vi "SA_EN_NON-STD_MEAS.vi"(6 "?":i32(ring) items=["NO", "YES"], 8 "error in":errorcluster {"code" format="%.0x"}, 11 "Session In":refnum<visa-resource-name>="TCPIP0::K-N90X0A-00005.local::hislip0::INSTR") -> (0 "error out":errorcluster {"code" format="%.0x"}, 3 "Session Out":refnum<visa-resource-name>)   [LabVIEW 2018]
panel:
  out "concatenated string":string
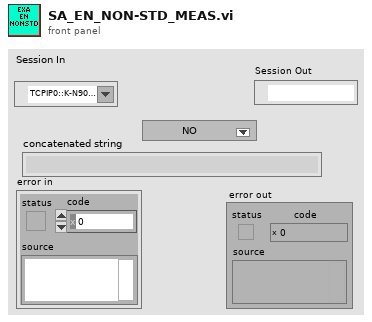
[diagram p1: front panel]
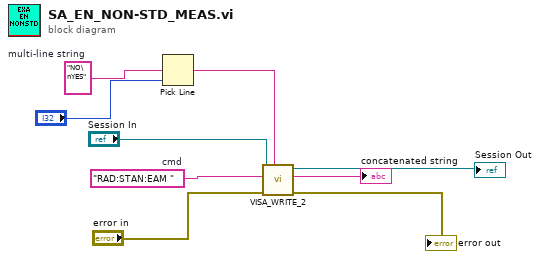
[diagram p0: block diagram]
diagram:
  w3 = "NO\nYES"  # multi-line string
  w9 = "RAD:STAN:EAM "  # cmd
  n1 = Pick Line(multi-line string=w3, line index="?") -> (output string=w4:string)  [unwired: 1 in]
  n2 = call "VISA_WRITE_2.vi"("Value (str)"=w4, "error in"="error in", "cmd"=w9, "Session In"="Session In") -> ("error out"=→"error out":errorcluster, "concatenated string"=→"concatenated string":string, "Session Out"=→"Session Out":refnum<visa-resource-name>)  [unwired: 5 in]
